vi "ZE_Recorder_CreateHeader.vi"(8 "Sampling Rate":dbl, 9 "No Samples":i32, 10 "Channel Array":T1 {"Terminal" items=["Default"=-1, "RSE"=10083, "NRSE"=10078, "Differential"=10106, "Pseudodifferential"=12529]}, 11 "Header Cluster":T5) -> (0 "TDMS propValues":string[](array[string]), 1 "TDMS properties":string[](array[string]), 3 "Header out":string)   [LabVIEW 2025, in "ZE_Recorder.lvlib"]
doc: "ZE_Recorder_CreateHeader.vi\n----------------------------------------------\nThe VI creates a file header for a CSV or TDMS file containing the relevant information about the measurement parameters\n\nInputs:\n---------------------\n- Sampling Rate : DBL; \n- Sampling Rate : I32; \n- Channel Array : 1DArrayOfCluster; \n- Header Cluster : Cluster; \n\nOutputs:\n---------------------\n- TDMS propValues : 1DArrayOfString; \n- TDMS properties : 1DArrayOfString; \n- Header out : String; \n\n----------------------------------------------\n02.06.2016\nZühlke Engineering AG\nCH-8952 Schlieren\nwww.zuehlke.com\n\nZE_ClusterToHeader.vi\n----------------------------------------------\nCreates a file header from the provided Information\n\nInputs:\n---------------------\n- Channel Array : 1DArrayOfCluster; \n- Header Cluster : Cluster; \n\nOutputs:\n---------------------\n- Header out : String; \n\n----------------------------------------------\n27.05.2016\nZühlke Engineering AG\nCH-8952 Schlieren\nwww.zuehlke.com"
uses:
  ZE_Recorder.lvlib
  ZE_Recorder_Header.ctl
  ZE_Recorder_ChannelCluster.ctl
  ChannelCluster.ctl
  ZE_Recorder_Units.ctl
  Temperature.ctl
panel:
  # "Connector Pane"
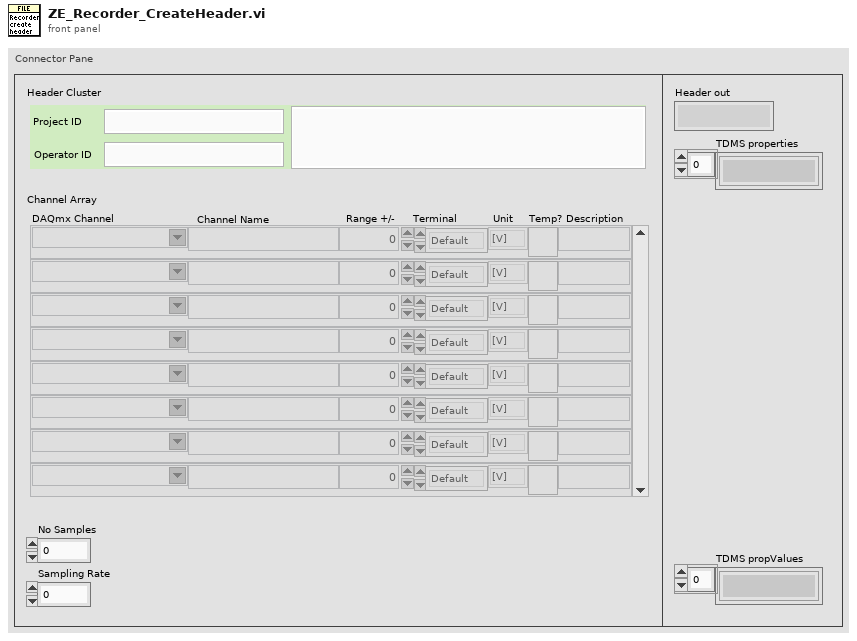
[diagram p1: front panel]
types:
  T1 = typedef "ZE_Recorder.lvlib/ZE_Recorder_ChannelCluster.ctl" = T2[]
  T2 = typedef "ZE_Recorder.lvlib/ChannelCluster.ctl" = cluster{"physical channel":tag, "channel name":string, "Range":dbl, "Terminal":i32, "Unit":T3, "isTemp":T4, "Description":string}
  T3 = typedef "ZE_Recorder.lvlib/ZE_Recorder_Units.ctl" = enum16{"[V]", "[A]", "[F]", "[H]", "[°C]", "[ml/s]", "[m/s]", "[bar]", "[%]", "[N]", "[?]"}
  T4 = typedef "ZE_Recorder.lvlib/Temperature.ctl" = bool
  T5 = typedef "ZE_Recorder.lvlib/ZE_Recorder_Header.ctl" = cluster{"Project":string, "Operator ID":string, "Description":string}
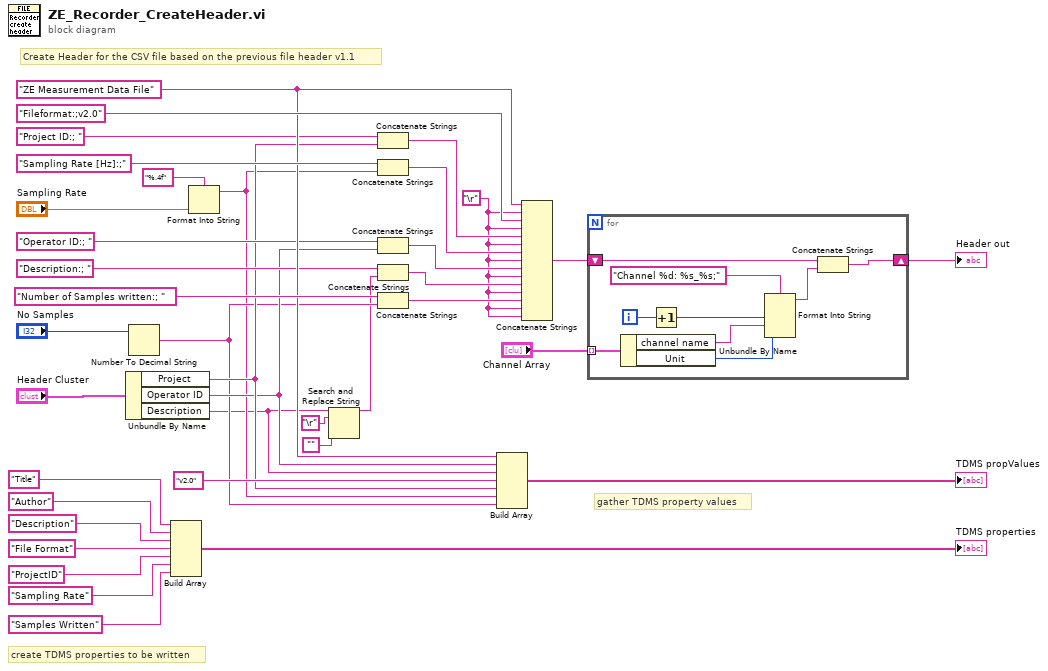
[diagram p0: block diagram]
diagram:
  w23 = "ZE Measurement Data File" ("string")
  w25 = "\r"
  # "gather TDMS property values"
  # "create TDMS properties to be written"
  # "Create Header for the CSV file based on the previous file header v1.1"
  n1 = Unbundle By Name("Header Cluster") -> ("Project"=w14:string, "Operator ID"=w13:string, "Description"=w2:string)
  n2 = Number To Decimal String(number="No Samples") -> (decimal integer string=w11:string)  [unwired: 1 in]
  n3 = Build Array("Title" ("string"), "Author" ("string"), "Description" ("string"), "File Format" ("string"), "ProjectID" ("element"), "Sampling Rate" ("element"), "Samples Written" ("element")) -> (→"TDMS properties":string[])
  n4 = Format Into String(format string="%.4f", "Sampling Rate") -> (resulting string=w5:string)  [unwired: 2 in, 1 out]
  n5 = Search and Replace String(input string=w2, search string="\r", replace string="" ("replace string (\"\")")) -> (result string=w1:string)  [unwired: 5 in, 3 out]
  n6 = Concatenate Strings("Project ID:; ", w14) -> (w31:string)
  n7 = Concatenate Strings("Sampling Rate [Hz]:;" ("string"), w5) -> (w26:string)
  n8 = Concatenate Strings("Operator ID:; ", w13) -> (w37:string)
  n9 = Concatenate Strings("Description:; ", w1) -> (w36:string)
  n10 = Concatenate Strings("Number of Samples written:; ", w11) -> (w27:string)
  n11 = Build Array(w23, w13, w2, "v2.0" ("element"), w14, w5, w11) -> (→"TDMS propValues":string[])
  n12 = Concatenate Strings(w23, w25, "Fileformat:;v2.0" ("string"), w25, w31, w25, w26, w25, w37, w25, w36, w25, w27, w25, w25) -> (w35:string)
  n13 = for {
    shift-right: [w40] -> w33
    shift-left: w35 -> [w42]
    tunnel: "Channel Array" -> [w47] mode=indexing
    i -> [w46]
    n14 = Unbundle By Name(w47) -> ("channel name"=w43:string, "Unit"=w39:T3)
    n15 = Increment(x=w46) -> (x+1=w44:i32)
    n16 = Format Into String(format string="Channel %d: %s_%s;" ("string"), w44, w43, w39) -> (resulting string=w41:string)  [unwired: 2 in, 1 out]
    n17 = Concatenate Strings(w42, w41) -> (w40:string)
  }
  "Header out" <- w33
